vi "Set Roller Orientation_Multiple.vi"(8 "error in (no error)":errorcluster, 10 "roller orientations":T1[](array[typedef]) items=["Left", "Right"], 11 "mecanum wheels in":refnum<class "NI_Robotics_Mecanum Wheel.lvclass">[](array[class])) -> (0 "error out":errorcluster, 3 "mecanum wheels out":refnum<class "NI_Robotics_Mecanum Wheel.lvclass">[](array[class]))   [LabVIEW 2017, in "NI_Robotics_Mecanum Wheel.lvclass"]
uses:
  <vilib>/robotics/Steering/Mecanum Wheel/NI_Robotics_Mecanum Wheel.lvclass
  <vilib>/robotics/Steering/Mecanum Wheel/Roller Orientation.ctl
  <vilib>/robotics/Steering/Mecanum Wheel/NI_Robotics_Mecanum Wheel.lvclass/NI_Robotics_Mecanum Wheel.ctl
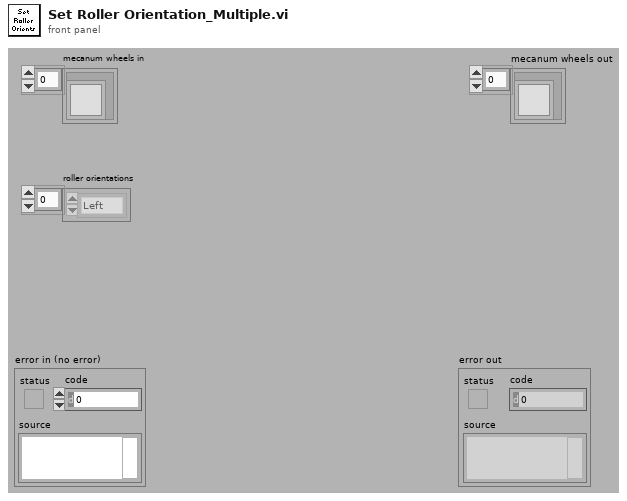
[diagram p1: front panel]
types:
  T1 = typedef "NI_Robotics_Mecanum Wheel.lvclass/Roller Orientation.ctl" = u16
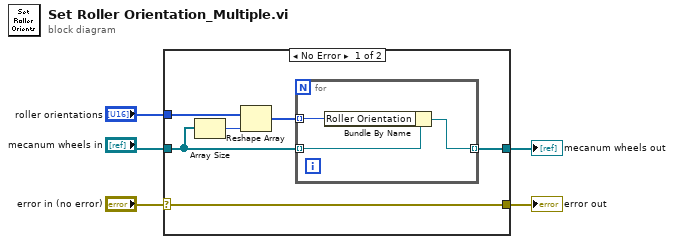
[diagram p0: block diagram]
diagram:
  n1 = case shown="No Error" "error in (no error)" {
    selector: "error in (no error)" -> [w11 w16]
    tunnel: [w11 w16] -> w4
    tunnel: "mecanum wheels in" -> [w8 w15]
    tunnel: "roller orientations" -> [w9 _]
    tunnel: [w6 w15] -> w1
    frame No Error {
      n2 = Array Size(array=w8) -> (size(s)=w10:i32)
      n3 = Reshape Array(w9, w10) -> (w7:T1[])
      n4 = for {
        tunnel: w8 -> [w14] mode=indexing
        tunnel: w7 -> [w13] mode=indexing
        tunnel: [w12] -> w6 mode=indexing
        n5 = Bundle By Name(cluster=w14, "Roller Orientation"=w13) -> (w12:refnum<class "NI_Robotics_Mecanum Wheel.lvclass">)
      }
    }
    frame Error {
    }
  }
  "error out" <- w4
  "mecanum wheels out" <- w1
